vi "Save Digital Patterns.vi"(8 "error in (no error)":errorcluster, 10 "Patterns":T1[](array[typedef]), 11 "Item Ref in":T5 format="%.0x") -> (0 "error out":errorcluster)   [LabVIEW 2013, in "Engine Simulation Toolkit System Explorer.lvlib"]
uses:
  Engine Simulation Toolkit System Explorer.lvlib
  <vilib>/NI Veristand/Custom Device API/Custom Device Item Ref.ctl
  Digital Pattern.ctl
  Digital Pattern Base.ctl
  Digital Pattern Remove Edge.ctl
  Digital Pattern Add Pulse.ctl
  Shared/Properties.vi
  <vilib>/NI Veristand/Custom Device API/Set Item Property (String).vi
  <vilib>/NI Veristand/Custom Device API/Set Item Property (Double).vi
  <vilib>/NI Veristand/Custom Device API/Set Item Property (U16).vi
  <vilib>/NI Veristand/Custom Device API/Set Item Property (Boolean).vi
  Shared/Engine Simulation Toolkit Shared.lvlib
  <vilib>/NI Veristand/Custom Device API/Custom Device API.lvlib
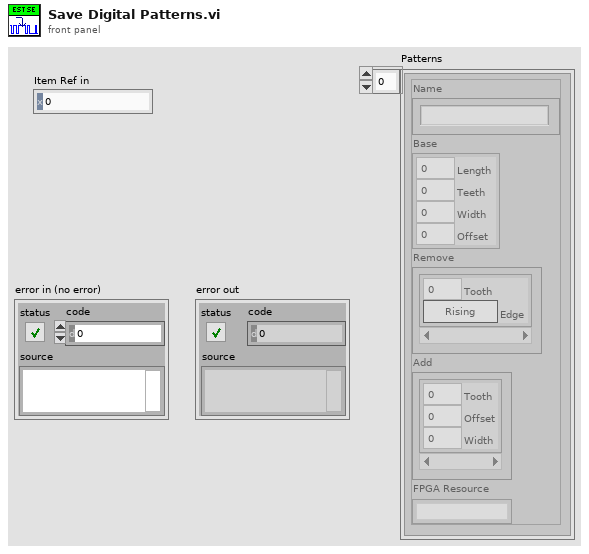
[diagram p1: front panel]
types:
  T1 = typedef "Engine Simulation Toolkit System Explorer.lvlib/Digital Pattern.ctl" = cluster{"Name":string, "Base":T2, "Remove":T3[], "Add":T4[], "FPGA Resource":string}
  T2 = typedef "Engine Simulation Toolkit System Explorer.lvlib/Digital Pattern Base.ctl" = cluster{"Length":dbl, "Teeth":u16, "Width":dbl, "Offset":dbl}
  T3 = typedef "Engine Simulation Toolkit System Explorer.lvlib/Digital Pattern Remove Edge.ctl" = cluster{"Tooth":u16, "Edge":bool}
  T4 = typedef "Engine Simulation Toolkit System Explorer.lvlib/Digital Pattern Add Pulse.ctl" = cluster{"Tooth":u16, "Offset":dbl, "Width":dbl}
  T5 = typedef "Custom Device API.lvlib/Custom Device Item Ref.ctl" = u64
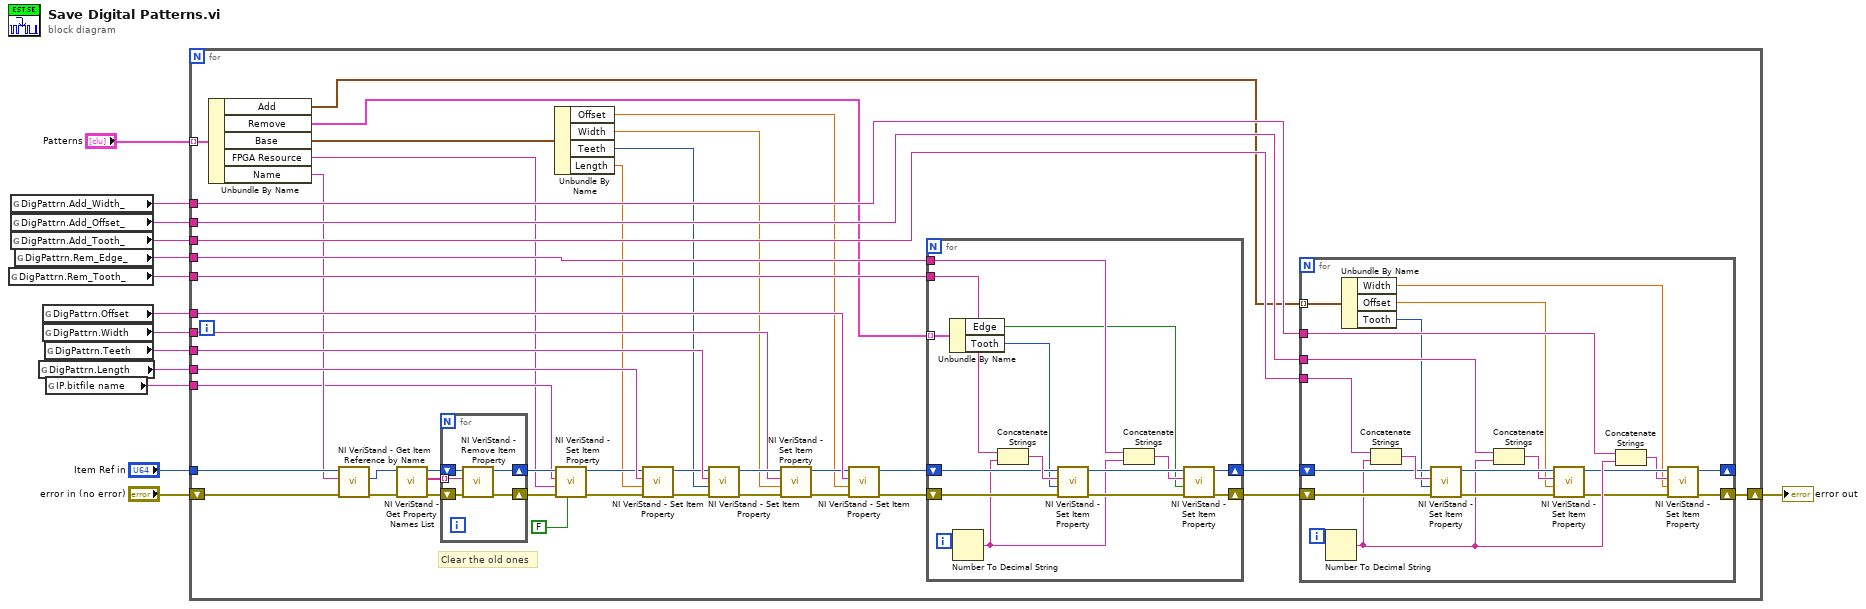
[diagram p0: block diagram]
diagram:
  n1 = global read "Properties.vi" "DigPattrn.Rem_Tooth_"() -> (w8:string)
  n2 = global read "Properties.vi" "DigPattrn.Add_Width_"() -> (w6:string)
  n3 = global read "Properties.vi" "DigPattrn.Add_Offset_"() -> (w5:string)
  n4 = global read "Properties.vi" "DigPattrn.Add_Tooth_"() -> (w4:string)
  n5 = global read "Properties.vi" "DigPattrn.Rem_Edge_"() -> (w7:string)
  n6 = global read "Properties.vi" "DigPattrn.Length"() -> (w12:string)
  n7 = global read "Properties.vi" "DigPattrn.Offset"() -> (w9:string)
  n8 = global read "Properties.vi" "DigPattrn.Width"() -> (w10:string)
  n9 = global read "Properties.vi" "DigPattrn.Teeth"() -> (w11:string)
  n10 = global read "Properties.vi" "IP.bitfile name"() -> (w1:string)
  n11 = for {
    shift-right: [w49] -> w13
    shift-left: "error in (no error)" -> [w57]
    tunnel: w12 -> [w56]
    tunnel: w11 -> [w55]
    tunnel: w10 -> [w38]
    tunnel: w9 -> [w54]
    tunnel: w8 -> [w53]
    tunnel: w7 -> [w52]
    tunnel: w4 -> [w50]
    tunnel: w5 -> [w37]
    tunnel: w6 -> [w51]
    tunnel: "Item Ref in" -> [w34]
    tunnel: "Patterns" -> [w36] mode=indexing
    tunnel: w1 -> [w23]
    # "Clear the old ones"
    n12 = Unbundle By Name(w36) -> ("Add"=w16:T4[], "Remove"=w17:T3[], "Base"=w32:T2, "FPGA Resource"=w22:string, "Name"=w33:string)
    n13 = call <vilib>:"NI VeriStand - Get Item Reference by Name.vi"("error in (no error)"=w57, "Item Name"=w33, "Parent Ref in"=w34) -> ("error out"=w35:errorcluster, "Item Ref"=w30:T5)  [unwired: 5 in, 2 out]
    n14 = call <vilib>:"NI VeriStand - Get Property Names List.vi"("error in (no error)"=w35, "Item Ref in"=w30) -> ("error out"=w31:errorcluster, "Property Names"=w27:string[], "Item Ref out"=w28:T5)  [unwired: 7 in]
    n15 = for {
      tunnel: w27 -> [w93] mode=indexing
      shift-right: [w94] -> w25
      shift-left: w28 -> [w95]
      shift-right: [w96] -> w29
      shift-left: w31 -> [w97]
      n16 = call <vilib>:"NI VeriStand - Remove Item Property.vi"("error in (no error)"=w97, "Property Name"=w93, "Item Ref in"=w95) -> ("error out"=w96:errorcluster, "Item Ref out"=w94:T5)  [unwired: 6 in, 1 out]
    }
    n17 = Unbundle By Name(w32) -> ("Offset"=w18:dbl, "Width"=w19:dbl, "Teeth"=w20:u16, "Length"=w21:dbl)
    n18 = call-poly <vilib>:"NI VeriStand - Set Item Property.vi"("Binary String (T)"=FALSE, "error in (no error)"=w29, "Value"=w22, "Property Name"=w23, "Item Ref in"=w25) -> ("error out"=w26:errorcluster, "Item Ref out"=w24:T5)  [unwired: 4 in, 1 out]
    n19 = call-poly <vilib>:"NI VeriStand - Set Item Property.vi"("error in (no error)"=w26, "Value"=w21, "Property Name"=w56, "Item Ref in"=w24) -> ("error out"=w47:errorcluster, "Item Ref out"=w48:T5)  [unwired: 5 in, 1 out]
    n20 = call-poly <vilib>:"NI VeriStand - Set Item Property.vi"("error in (no error)"=w47, "Value"=w20, "Property Name"=w55, "Item Ref in"=w48) -> ("error out"=w45:errorcluster, "Item Ref out"=w46:T5)  [unwired: 5 in, 1 out]
    n21 = call-poly <vilib>:"NI VeriStand - Set Item Property.vi"("error in (no error)"=w45, "Value"=w19, "Property Name"=w38, "Item Ref in"=w46) -> ("error out"=w43:errorcluster, "Item Ref out"=w44:T5)  [unwired: 5 in, 1 out]
    n22 = call-poly <vilib>:"NI VeriStand - Set Item Property.vi"("error in (no error)"=w43, "Value"=w18, "Property Name"=w54, "Item Ref in"=w44) -> ("error out"=w39:errorcluster, "Item Ref out"=w40:T5)  [unwired: 5 in, 1 out]
    n23 = for {
      shift-right: [w82] -> w41
      shift-left: w39 -> [w90]
      shift-right: [w83] -> w42
      shift-left: w40 -> [w91]
      tunnel: w52 -> [w86]
      tunnel: w53 -> [w84]
      tunnel: w17 -> [w80] mode=indexing
      i -> [w89]
      n24 = Unbundle By Name(w80) -> ("Edge"=w78:bool, "Tooth"=w79:u16)
      n25 = Number To Decimal String(number=w89) -> (decimal integer string=w85:string)  [unwired: 1 in]
      n26 = Concatenate Strings(w84, w85) -> (w92:string)
      n27 = call-poly <vilib>:"NI VeriStand - Set Item Property.vi"("error in (no error)"=w90, "Value"=w79, "Property Name"=w92, "Item Ref in"=w91) -> ("error out"=w88:errorcluster, "Item Ref out"=w87:T5)  [unwired: 5 in, 1 out]
      n28 = Concatenate Strings(w86, w85) -> (w81:string)
      n29 = call-poly <vilib>:"NI VeriStand - Set Item Property.vi"("error in (no error)"=w88, "Value"=w78, "Property Name"=w81, "Item Ref in"=w87) -> ("error out"=w82:errorcluster, "Item Ref out"=w83:T5)  [unwired: 5 in, 1 out]
    }
    n30 = for {
      shift-right: [w67] -> w49
      shift-left: w41 -> [w75]
      shift-right: [w68] -> _
      shift-left: w42 -> [w76]
      tunnel: w37 -> [w71]
      tunnel: w50 -> [w69]
      tunnel: w51 -> [w66]
      tunnel: w16 -> [w61] mode=indexing
      i -> [w74]
      n31 = Number To Decimal String(number=w74) -> (decimal integer string=w70:string)  [unwired: 1 in]
      n32 = Unbundle By Name(w61) -> ("Width"=w58:dbl, "Offset"=w59:dbl, "Tooth"=w60:u16)
      n33 = Concatenate Strings(w69, w70) -> (w77:string)
      n34 = call-poly <vilib>:"NI VeriStand - Set Item Property.vi"("error in (no error)"=w75, "Value"=w60, "Property Name"=w77, "Item Ref in"=w76) -> ("error out"=w73:errorcluster, "Item Ref out"=w72:T5)  [unwired: 5 in, 1 out]
      n35 = Concatenate Strings(w71, w70) -> (w65:string)
      n36 = call-poly <vilib>:"NI VeriStand - Set Item Property.vi"("error in (no error)"=w73, "Value"=w59, "Property Name"=w65, "Item Ref in"=w72) -> ("error out"=w63:errorcluster, "Item Ref out"=w64:T5)  [unwired: 5 in, 1 out]
      n37 = Concatenate Strings(w66, w70) -> (w62:string)
      n38 = call-poly <vilib>:"NI VeriStand - Set Item Property.vi"("error in (no error)"=w63, "Value"=w58, "Property Name"=w62, "Item Ref in"=w64) -> ("error out"=w67:errorcluster, "Item Ref out"=w68:T5)  [unwired: 5 in, 1 out]
    }
  }
  "error out" <- w13
